vi "ConvertLineStrToLineCnt.vi"(11 "Line Str":string="LGE Part No\nDate\nSerial\nFuse Barcoder\nToque1 Value\nToque2 Value\nRevision No\nMini Register Barcode\nGM Part Number\nVVPS Number\nDUNS Number") -> (2 "Arr String":string[](array[string]), 3 "Line Cnt":i32)   [LabVIEW 2018, in "Library-DataConvert.lvlib"]
uses:
  Library-DataConvert.lvlib
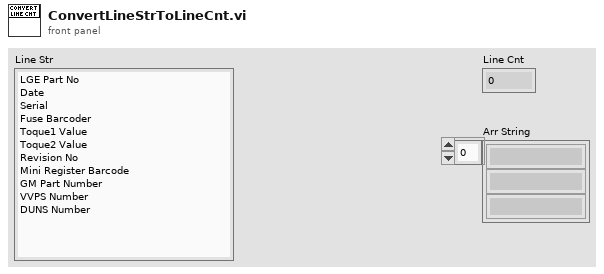
[diagram p1: front panel]
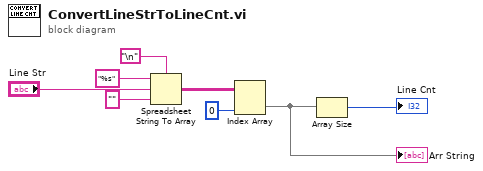
[diagram p0: block diagram]
diagram:
  n1 = Spreadsheet String To Array(delimiter (Tab)="\n", format string="%s" ("포맷 문자열"), spreadsheet string="Line Str", array type (2D Dbl)="") -> (array=w4:string[][])
  n2 = Index Array(array=w4, index (col)=0 ("비활성화된 인덱스 (열)")) -> (element=w2:string[])  [unwired: 1 in]
  "Arr String" <- w2
  n3 = Array Size(array=w2) -> (size(s)=→"Line Cnt":i32)
